vi "Find Tests - When Project Is Valid - Returns No Error.vi"() -> ()   [LabVIEW 2017, in "LVUnit Test Discoverer.Tests.lvlib"]
uses:
  LVUnit Test Discoverer.Tests.lvlib
  LVUnit Test Discoverer/LVUnit Test Discoverer.lvclass
  Assertion/Assertion.lvlib
panel:
  out "error out":errorcluster
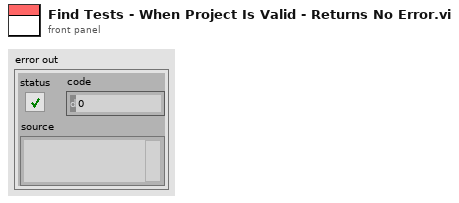
[diagram p1: front panel]
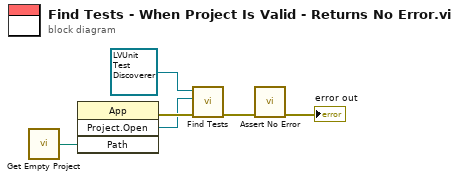
[diagram p0: block diagram]
diagram:
  n1 = call "Get Empty Project.vi"() -> ("Project File"=w3:path)  [unwired: 2 in]
  n2 = invoke class="App" method="Project.Open"("Path"=w3) -> (error out=w2:errorcluster, "Project:Open"=w1:refnum<vi>)  [unwired: 3 in, 2 out]
  n3 = call-dynamic "Find Tests.vi"("error in (no error)"=w2, "Project Refnum"=w1, "LVUnit Test Discoverer in"=refnum<class "LVUnit Test Discoverer.lvclass"> refnum ("LVUnit Test Discoverer")) -> ("error out"=w5:errorcluster)  [unwired: 6 in, 2 out]
  n4 = call "Assert No Error.vi"("error in (no error)"=w5) -> ("error out"=→"error out":errorcluster)  [unwired: 10 in]
